vi "Part 2.vi"(11 "Input":string) -> (3 "Output":i64)   [LabVIEW 2021]
uses:
  <userlib>/_OpenG.lib/string/string.llb/Convert EOLs (String)__ogtk.vi
  <vilib>/regexp/Match Regular Expression.xnode
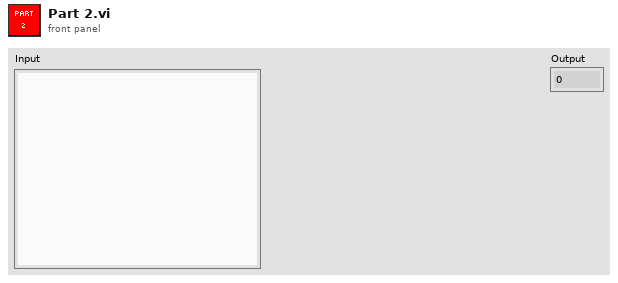
[diagram p1: front panel]
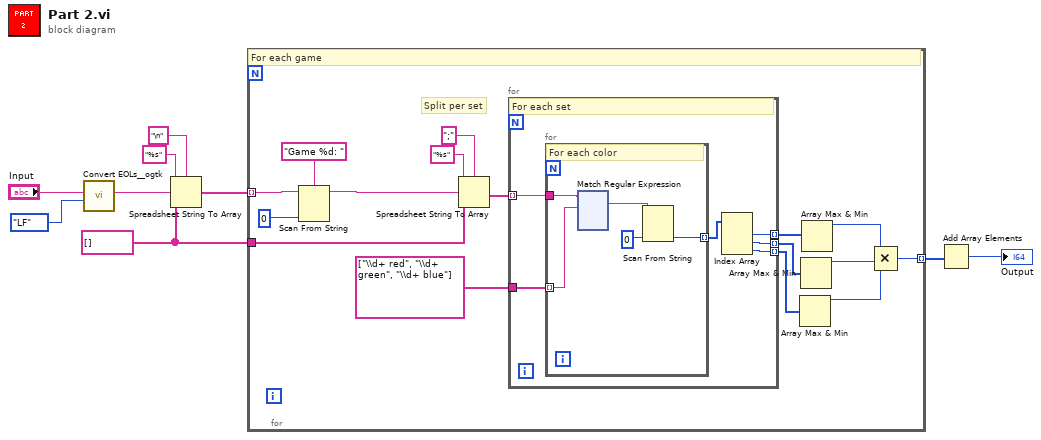
[diagram p0: block diagram]
diagram:
  w3 = string[] []
  n1 = call-poly <userlib>:"Convert EOLs__ogtk.vi"("Convert to:"=enum16{"CR", "LF", "CRLF"}."LF", "String in"="Input") -> ("String out"=w6:string)  [unwired: 9 in]
  n2 = Spreadsheet String To Array(delimiter (Tab)="\n", format string="%s", spreadsheet string=w6, array type (2D Dbl)=w3) -> (array=w4:string[])
  n3 = for {
    tunnel: w4 -> [w25] mode=indexing
    tunnel: w3 -> [w17]
    tunnel: [w10] -> w2 mode=indexing
    # "Split per set"
    # "For each game"
    n4 = Scan From String(format string="Game %d: ", input string=w25, default 1=0) -> (remaining string=w19:string)  [unwired: 3 in, 2 out]
    n5 = Spreadsheet String To Array(delimiter (Tab)=";", format string="%s", spreadsheet string=w19, array type (2D Dbl)=w17) -> (array=w18:string[])
    n6 = for {
      tunnel: string[] ["\\d+ red", "\\d+ green", "\\d+ blue"] -> [w31]
      tunnel: w18 -> [w30] mode=indexing
      tunnel: [w28] -> w16 mode=indexing
      tunnel: [w27] -> w15 mode=indexing
      tunnel: [w26] -> w14 mode=indexing
      # "For each set"
      n7 = for {
        tunnel: w30 -> [w36]
        tunnel: w31 -> [w33] mode=indexing
        tunnel: [w32] -> w29 mode=indexing
        # "For each color"
        n8 = xnode "Match Regular Expression"("input string"=w36, "regular expression"=w33) -> ("whole match"=w35:string)  [unwired: 4 in, 4 out]
        n9 = Scan From String(input string=w35, default 1=0) -> (output 1=w32:i32)  [unwired: 3 in, 3 out]
      }
      n10 = Index Array(array=w29) -> (element #1=w28:i32, element #2=w27:i32, element #3=w26:i32)  [unwired: 3 in]
    }
    n11 = Array Max & Min(array=w14) -> (max value=w11:i32)  [unwired: 3 out]
    n12 = Array Max & Min(array=w15) -> (max value=w12:i32)  [unwired: 3 out]
    n13 = Array Max & Min(array=w16) -> (max value=w13:i32)  [unwired: 3 out]
    n14 = Compound Arithmetic op=MULTIPLY(w13, w12, w11) -> (w10:i32)
  }
  n15 = Add Array Elements(numeric array=w2) -> (sum=→"Output":i32)
